vi "CLC_GEN4_L2_InPhaseCal_mW.vi"() -> ()   [LabVIEW 2023, in "Clover_Cell.lvlib"]
uses:
  Clover_Cell.lvlib
  lib/Anritsu Signal Analyzer Series/Anritsu Signal Analyzer Series.lvlib
  lib/ELTA/ELTA.lvlib
panel:
  in  "Daul_Ch_Phase_Sweep":bool
  in  "SweepSwitch?":u16(ring) items=["NoSweep(Single)", "Sweep"]
  in  "SweepMode":u16(ring) items=["Phase", "Gain"]
  in  "Method":u16(ring)=1 items=["dBm"=1, "mW"=2]
  in  "Polarity":u16(ring) items=["V", "H"]
  in  "VISA resource name":refnum<visa-resource-name>="TCPIP0::192.168.100.230::inst0::INSTR"
  in  "CenterFreq(GHz)":dbl=27.0
  in  "AvgTimes":i32=3
  in  "Single_Ch_Phase_Sweep":bool
  in  "TRXmode":u16(ring)=1 items=["Rx"=2, "Tx"=1]
  out "GainStep":i32=63
  out "PhaseStep":i32=63
  out "Channel":i32=63
  out "Total mW":dbl format="%.7f"
  out "Total dBm":dbl format="%.7f"
  out "Ref. mW":dbl format="%.7f"
  out "Ref. dBm":dbl format="%.7f"
  out "Main mW":dbl format="%.7f"
  out "Main dBm":dbl format="%.7f"
  out "Data":dbl[][](array[numeric])
  out "FileNAME_Single":string
  out "SA1":dbl[](graph)
  out "CurrentData":dbl[](array[numeric])
  out "Duration":dbl
  out "TotalTime":dbl format="%.2f"
  out "StopTime":timestamp=timestamp(3663835912.033212 s since 1904-01-01)
  out "FileNAME_Dual":string
  out "StartTime":timestamp=timestamp(3663835741.875155 s since 1904-01-01)
  out "TX/RX":u16=1
  out "error out":errorcluster
  out "output cluster":T1={"address"="192.168.100.111", "remote port or service name"=5025, "timeout ms (60000)"=10000}
  out "Operating \nChannel(s)":bool[][](array[boolean])
  out "OK?":bool
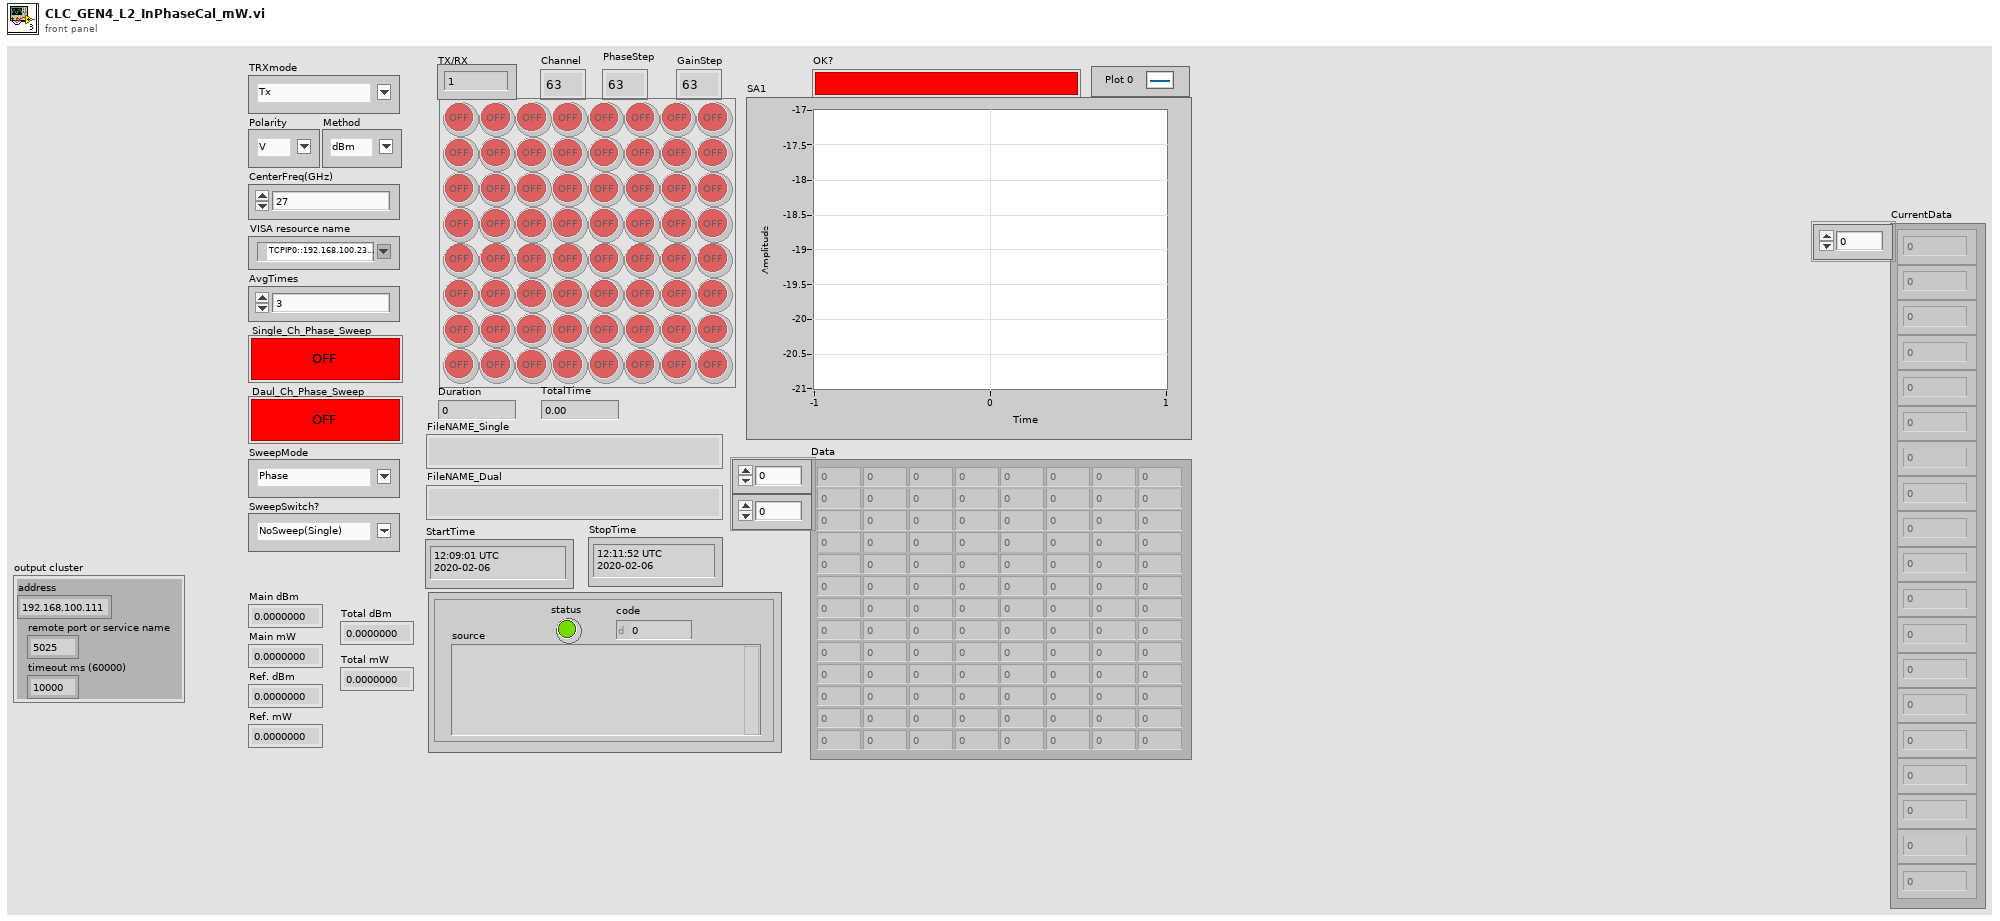
[diagram p1: front panel]
types:
  T1 = cluster{"address":string, "remote port or service name":u16, "timeout ms (60000)":i32}
  T2 = cluster{"Mode":u16, "Polarity":u16, "CH_ON/OFF":u16, "Channel":i32, "Gain":i32, "Phase":i32}
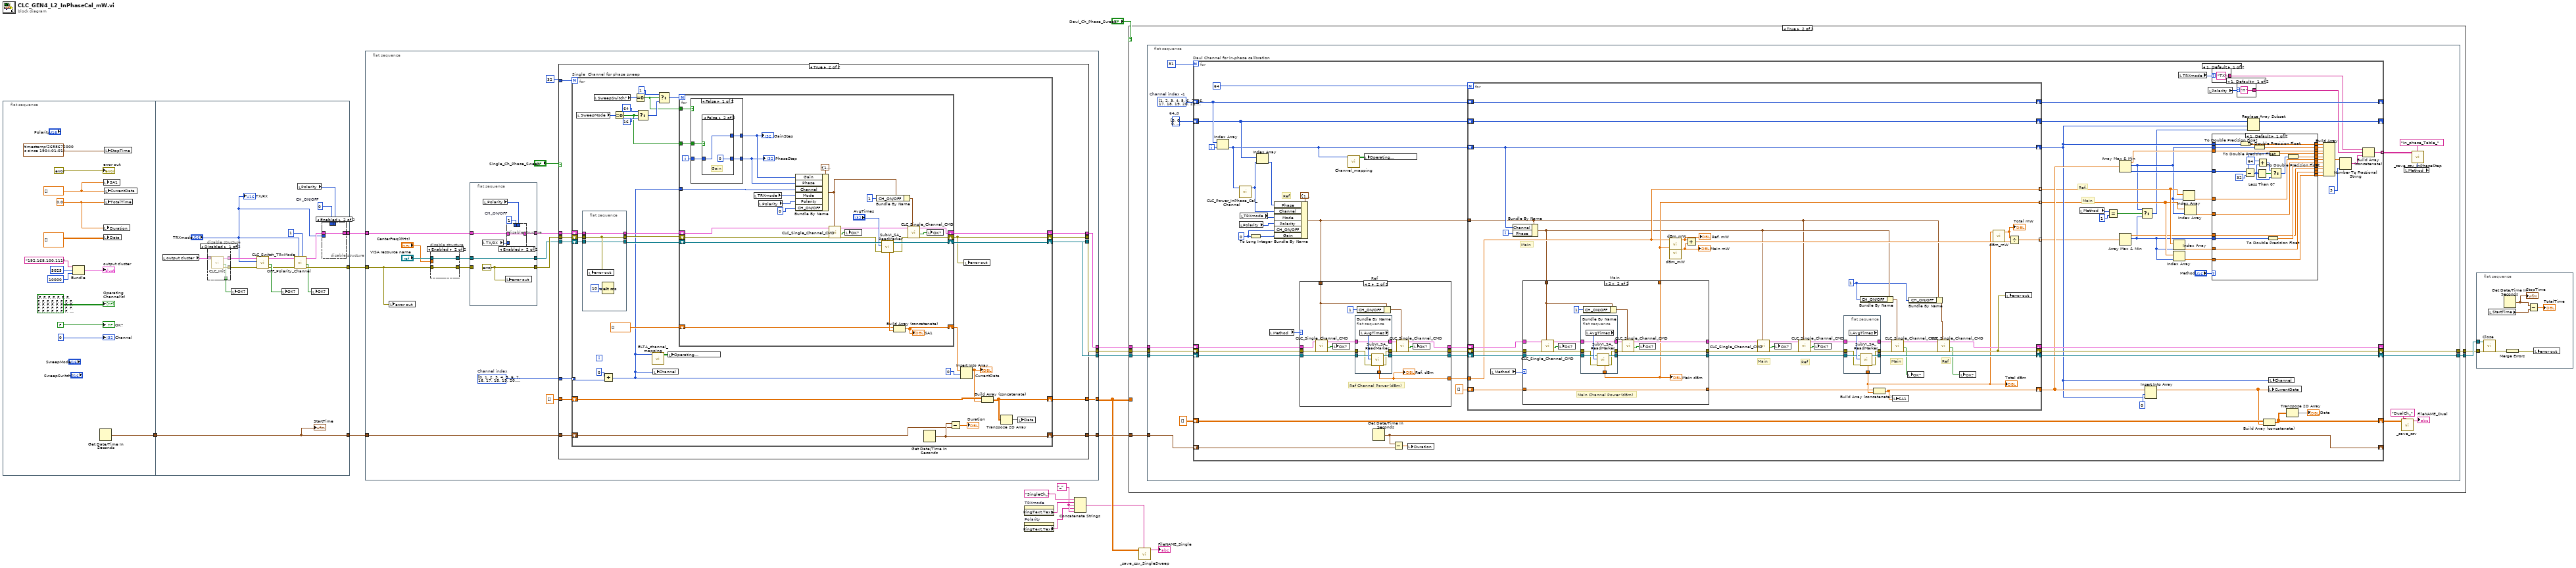
[diagram p0: block diagram]
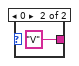
[diagram p3: hidden frame]
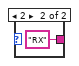
[diagram p4: hidden frame]
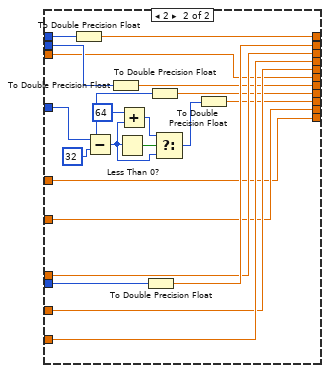
[diagram p5: hidden frame]
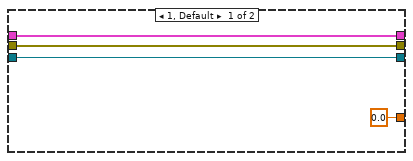
[diagram p6: hidden frame]
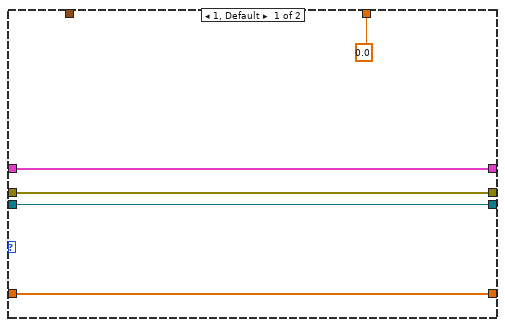
[diagram p7: hidden frame]
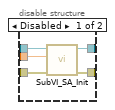
[diagram p8: hidden frame]
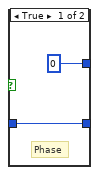
[diagram p10: hidden frame]
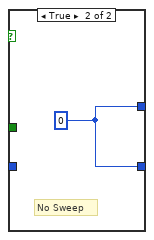
[diagram p11: hidden frame]
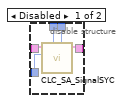
[diagram p12: hidden frame]
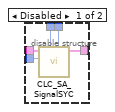
[diagram p13: hidden frame]
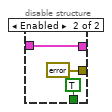
[diagram p14: hidden frame]
diagram:
  w2 = "_" ("delimiter (\\t)")
  n1 = flat-sequence {
    tunnel: [w19] -> w18
    tunnel: w18 -> [w35]
    tunnel: [w38] -> w9
    tunnel: [w42] -> w10
    tunnel: [w35] -> w17
    frame #0 {
      w23 = dbl[] []
      w26 = 0.0 ("TotalTime")
      n2 = Bundle("address"="192.168.100.111", "remote port or service name"=u16 5025, "timeout ms (60000)"=10000) -> (→"output cluster":T1)  [unwired: 1 in]
      n3 = Get Date/Time In Seconds() -> (seconds since 1Jan1904=w19:timestamp)
      n4 = local write "SA1"(w23) -> ()
      n5 = local write "Duration"(w26) -> ()
      n6 = local write "Data"(dbl[][] []) -> ()
      n7 = local write "StopTime"(timestamp(2658672000.001 s since 1904-01-01) ("StopTime")) -> ()
      n8 = local write "CurrentData"(w23) -> ()
      n9 = local write "TotalTime"(w26) -> ()
      "error out" <- errorcluster {"status"=FALSE, "code"=0, "source"=""} ("error out")
      "Operating \nChannel(s)" <- bool[][] [[FALSE, FALSE, FALSE, FALSE, FALSE, FALSE, FALSE, FALSE], [FALSE, FALSE, FALSE, FALSE, FALSE, FALSE, FALSE, FALSE], [FALSE, FALSE, FALSE, FALSE, FALSE, FALSE, FALSE, FALSE], [FALSE, FALSE, FALSE, FALSE, FALSE, FALSE, FALSE, FALSE], [FALSE, FALSE, FALSE, FALSE, FALSE, FALSE, FALSE, FALSE], [FALSE, FALSE, FALSE, FALSE, FALSE, FALSE, FALSE, FALSE], [FALSE, FALSE, FALSE, FALSE, FALSE, FALSE, FALSE, FALSE], [FALSE, FALSE, FALSE, FALSE, FALSE, FALSE, FALSE, FALSE]] ("Operating \nChannel(s)")
      "Channel" <- 0 ("Channel")
      "OK?" <- FALSE ("OK?")
    }
    frame #1 {
      w37 = u16 0  # CH_ON/OFF
      n10 = local read "output cluster"() -> (w47:T1)
      n11 = disable-structure shown="Disabled" {
        disable-tunnel: w47 -> [w57 w60]
        disable-tunnel: [w56 w60] -> w46
        disable-tunnel: [w55 errorcluster {"status"=FALSE, "code"=0, "source"=""} ("error in (no error)")] -> w44
        disable-tunnel: [w54 TRUE ("OK?")] -> w36
        frame Disabled {
          n12 = call "CLC_Init.vi"("TCPIPin"=w57) -> ("error out"=w55:errorcluster, "Status"=w54:bool, "TCPIPin 2"=w56:T1)  [unwired: 8 in]
        }
        frame Enabled {
        }
      }
      n13 = local write "OK?"(w36) -> ()
      n14 = call "CLC_Switch_TRxMode.vi"("error in (no error)"=w44, "Text Ring"="TRXmode", "TCPIPin"=w46) -> ("error out"=w43:errorcluster, "OK?"=w45:bool, "TCPIPin 2"=w41:T1)  [unwired: 6 in]
      n15 = local write "OK?"(w45) -> ()
      n16 = call "OFF_Polarity_Channel.vi"("CH_ON:0/OFF:1"=u16 1, "Mode"="TRXmode", "error in"=w43, "TCPIPin"=w41) -> ("error out"=w42:errorcluster, "OK?"=w40:bool, "TCPIPout"=w39:T1)  [unwired: 5 in]
      n17 = local read "Polarity"() -> (w33:u16)
      n18 = local write "OK?"(w40) -> ()
      n19 = disable-structure shown="Enabled" {
        disable-tunnel: w39 -> [w52 w53]
        disable-tunnel: [w51 w53] -> w38
        disable-tunnel: w37 -> [w50 _]
        disable-tunnel: w33 -> [w49 _]
        disable-tunnel: "TRXmode" -> [w48 _]
        frame Disabled {
          n20 = call "CLC_SA_SignalSYC.vi"("Polarity"=w49, "CH_ON/OFF"=w50, "Mode"=w48, "TCPIPin"=w52) -> ("TCPIPout"=w51:T1)  [unwired: 7 in]
        }
        frame Enabled {
        }
      }
      "StartTime" <- w35
      "TX/RX" <- "TRXmode"
    }
  }
  n21 = flat-sequence {
    tunnel: w17 -> [w77]
    tunnel: [w76] -> w16
    tunnel: [w75] -> w15
    tunnel: [w74] -> w14
    tunnel: [w73] -> w11
    tunnel: w10 -> [w71]
    tunnel: w9 -> [w66]
    tunnel: [w61] -> w6
    frame #0 {
      w68 = i32[] [0, 1, 2, 3, 4, 5, 6, 7, 16, 17, 18, 19, 20, 21, 22, 23, 32, 33, 34, 35, 36, 37, 38, 39, 48, 49, 50, 51, 52, 53, 54, 55]  # Channel index
      n22 = local write "error out"(w71) -> ()
      n23 = disable-structure shown="Enabled" {
        disable-tunnel: "VISA resource name" -> [w84 w86]
        disable-tunnel: [w83 w85] -> w72
        disable-tunnel: w71 -> [w82 w85]
        disable-tunnel: "CenterFreq(GHz)" -> [w81 _]
        disable-tunnel: [w80 w86] -> w65
        frame Disabled {
          n24 = call "SubVI_SA_Init.vi"("error in (no error)"=w82, "CenterFreq(GHz) 2"=w81, "VISA resource name"=w84) -> ("error out 2"=w83:errorcluster, "VISA resource name out"=w80:refnum<visa-resource-name>)  [unwired: 6 in, 1 out]
        }
        frame Enabled {
        }
      }
      n25 = flat-sequence {
        tunnel: w72 -> [_]
        tunnel: [w177] -> w67
        tunnel: w66 -> [w182]
        tunnel: w65 -> [w183]
        tunnel: [w183] -> w64
        tunnel: [w181] -> w63
        frame #0 {
          w177 = errorcluster {"status"=FALSE, "code"=0, "source"=""} ("error in (no error)")
          w180 = u16 1  # CH_ON/OFF
          n26 = local read "TX/RX"() -> (w178:u16)
          n27 = local read "Polarity"() -> (w179:u16)
          n28 = local write "error out"(w177) -> ()
          n29 = disable-structure shown="Enabled" {
            disable-tunnel: w182 -> [w188 w189]
            disable-tunnel: [w187 w189] -> w181
            disable-tunnel: w180 -> [w186 _]
            disable-tunnel: w179 -> [w185 _]
            disable-tunnel: w178 -> [w184 _]
            frame Disabled {
              n30 = call "CLC_SA_SignalSYC.vi"("Polarity"=w185, "CH_ON/OFF"=w186, "Mode"=w184, "TCPIPin"=w188) -> ("TCPIPout"=w187:T1)  [unwired: 7 in]
            }
            frame Enabled {
            }
          }
        }
      }
      n31 = case shown="True" "Single_Ch_Phase_Sweep" {
        tunnel: [w88 w103] -> w61
        tunnel: 32 -> [_ w102]
        tunnel: w77 -> [w87 w101]
        tunnel: [w89 w100] -> w76
        tunnel: [w90 w99] -> w75
        tunnel: [w91 w98] -> w74
        tunnel: [w87 w97] -> w73
        tunnel: dbl[][] [] -> [w88 w96]
        tunnel: w68 -> [_ w95]
        tunnel: w67 -> [w90 w94]
        tunnel: w64 -> [w89 w93]
        tunnel: w63 -> [w91 w92]
        frame False {
        }
        frame True {
          n32 = for "Single  Channel for phase sweep" {
            N: w102 -> [_]
            shift-right: [w135] -> w98
            shift-left: w92 -> [w120]
            shift-right: [w130] -> w99
            shift-left: w94 -> [w122]
            shift-right: [w134] -> w100
            shift-left: w93 -> [w119]
            shift-right: [w128] -> w103
            shift-left: w96 -> [w129]
            shift-right: [w132] -> w97
            shift-left: w101 -> [w131]
            tunnel: w95 -> [w116] mode=indexing
            n33 = local read "SweepMode"() -> (w112:u16)
            n34 = flat-sequence {
              tunnel: [w137] -> w118
              tunnel: w122 -> [w138]
              tunnel: [w138] -> w121
              tunnel: w120 -> [w137]
              tunnel: w119 -> [w136]
              tunnel: [w136] -> w117
              frame #0 {
                n35 = local write "error out"(w138) -> ()
                n36 = Wait (ms)(milliseconds to wait=u32 10) -> ()  [unwired: 1 out]
              }
            }
            n37 = local read "SweepSwitch?"() -> (w111:u16)
            n38 = Add(x=0, y=w116) -> (x+y=w113:i32)
            n39 = Equal To 0?(x=w112) -> (x = 0?=w104:bool)
            n40 = Equal To 0?(x=w111) -> (x = 0?=w105:bool)
            n41 = Select(t=64, s=w104, f=16) -> (s? t:f=w106:i32)
            n42 = call "ELTA_channel_mapping.vi"("Channel IN"=w113) -> ("Operating \nChannel(s)"=w114:bool[][])  [unwired: 10 in]
            n43 = local write "Channel"(w113) -> ()
            n44 = Select(t=1, s=w105, f=w106) -> (s? t:f=w109:i32)
            n45 = local write "Operating \nChannel(s)"(w114) -> ()
            n46 = for {
              N: w109 -> [_]
              shift-right: [w149] -> w135
              shift-left: w118 -> [w159]
              shift-right: [w151] -> w130
              shift-left: w121 -> [w161]
              shift-right: [w166] -> w134
              shift-left: w117 -> [w167]
              shift-right: [w162] -> w127
              shift-left: dbl[] [] -> [w163]
              tunnel: w113 -> [w156]
              tunnel: w105 -> [w144]
              tunnel: w104 -> [w141]
              i -> [w140]
              n47 = case shown="False" w144 {
                tunnel: [w168 w176] -> w143
                tunnel: [w169 w176] -> w142
                tunnel: w141 -> [w171 _]
                tunnel: w140 -> [w170 _]
                frame False {
                  n48 = case shown="False" w171 {
                    tunnel: w170 -> [w173 w174]
                    tunnel: [w173 0] -> w169
                    tunnel: [0 w174] -> w168
                    frame True {
                      # "Phase"
                    }
                    frame False {
                      # "Gain"
                    }
                  }
                }
                frame True {
                  w176 = 0
                  # "No Sweep"
                }
              }
              "PhaseStep" <- w142
              "GainStep" <- w143
              n49 = local read "TRXmode"() -> (w155:u16)
              n50 = local read "Polarity"() -> (w154:u16)
              n51 = Bundle By Name(cluster=T2 {"Mode"=1, "Polarity"=1, "CH_ON/OFF"=1, "Channel"=0, "Gain"=0, "Phase"=0} ("Channel params"), "Gain"=w143, "Phase"=w142, "Channel"=w156, "Mode"=w155, "Polarity"=w154, "CH_ON/OFF"=u16 0) -> (w148:T2)
              n52 = call "CLC_Single_Channel_CMD.vi"("Channel params"=w148, "error in"=w161, "TCPIPin"=w159) -> ("error out"=w160:errorcluster, "OK?"=w157:bool, "TCPIPout"=w150:T1)  [unwired: 6 in]
              n53 = local write "OK?"(w157) -> ()
              n54 = Bundle By Name(cluster=w148, "CH_ON/OFF"=u16 1) -> (w146:T2)
              n55 = call "SubVI_SA_ReadMarker.vi"("error in (no error)"=w160, "AvgTimes"="AvgTimes", "VISA resource name"=w167) -> ("error out"=w152:errorcluster, "VISA resource name out"=w166:refnum<visa-resource-name>, "Marker Power"=w164:dbl)  [unwired: 5 in, 1 out]
              n56 = Build Array (concatenate)(w163, w164) -> (w162:dbl[])
              "SA1" <- w162
              n57 = call "CLC_Single_Channel_CMD.vi"("Channel params"=w146, "error in"=w152, "TCPIPin"=w150) -> ("error out"=w151:errorcluster, "OK?"=w145:bool, "TCPIPout"=w149:T1)  [unwired: 6 in]
              n58 = local write "OK?"(w145) -> ()
            }
            n59 = Get Date/Time In Seconds() -> (seconds since 1Jan1904=w132:timestamp)
            n60 = Subtract(x=w132, y=w131) -> (x-y=→"Duration":dbl)
            n61 = Insert Into Array(array=w127, index=0, new element=w113) -> (w124:dbl[])
            "CurrentData" <- w124
            n62 = local write "error out"(w130) -> ()
            n63 = Build Array (concatenate)(w129, w124) -> (w128:dbl[][])
            n64 = Transpose 2D Array(2D array=w128) -> (transposed array=w115:dbl[][])
            n65 = local write "Data"(w115) -> ()
          }
        }
      }
    }
  }
  n66 = property on="TRXmode" class="Ring (strict)"() -> ("RingText.Text"=w4:string)  [unwired: 2 in, 2 out]
  n67 = property on="Polarity" class="Ring (strict)"() -> ("RingText.Text"=w1:string)  [unwired: 2 in, 2 out]
  n68 = Concatenate Strings("SingleCh_" ("delimiter (\\t)"), w4, w2, w1, w2) -> (w3:string)
  n69 = case shown="True" "Daul_Ch_Phase_Sweep" {
    tunnel: w16 -> [w191 w197]
    tunnel: w15 -> [w190 w196]
    tunnel: w14 -> [_ w195]
    tunnel: [w191 w194] -> w13
    tunnel: [w190 w193] -> w12
    tunnel: w11 -> [_ w192]
    tunnel: w6 -> [_ _]
    frame False {
    }
    frame True {
      n70 = flat-sequence {
        tunnel: w197 -> [w212]
        tunnel: w196 -> [w211]
        tunnel: w195 -> [w210]
        tunnel: [w209] -> w194
        tunnel: [w208] -> w193
        tunnel: w192 -> [w207]
        frame #0 {
          w204 = i32[] [0, 0, 0, 0, 0, 0, 0, 0, 0, 0, 0, 0, 0, 0, 0, 0, 0, 0, 0, 0, 0, 0, 0, 0, 0, 0, 0, 0, 0, 0, 0, 0, 0, 0, 0, 0, 0, 0, 0, 0, 0, 0, 0, 0, 0, 0, 0, 0, 0, 0, 0, 0, 0, 0, 0, 0, 0, 0, 0, 0, 0, 0, 0, 0]  # 64_0
          w205 = i32[] [1, 2, 3, 4, 5, 6, 7, 16, 17, 18, 19, 20, 21, 22, 23, 32, 33, 34, 35, 36, 37, 38, 39, 48, 49, 50, 51, 52, 53, 54, 55]  # Channel index -1
          n71 = for "Daul Channel for in-phase calibration" {
            N: 31 -> [_]
            shift-right: [w288] -> _
            shift-left: w210 -> [w249]
            shift-right: [w285] -> w208
            shift-left: w211 -> [w253]
            shift-right: [w286] -> w209
            shift-left: w212 -> [w251]
            shift-right: [w280] -> w199
            shift-left: dbl[][] [] -> [w281]
            shift-right: [w284] -> _
            shift-left: w207 -> [w283]
            shift-right: [w271] -> _
            shift-left: w204 -> [w246]
            tunnel: [w214] -> w200 mode=indexing
            shift-right: [w273] -> _
            shift-left: w205 -> [w272]
            i -> [w274]
            w255 = u16 0 ("CH_ON/OFF")
            # "Main"
            # "Ref."
            # "Ref"
            n72 = Index Array(array=w272, index=w274) -> (element=w242:i32)
            n73 = call "CLC_Power_InPhase_Cal_Channel.vi"("Channel IN"=w242) -> ("Ref_Channel"=w241:i32)  [unwired: 8 in, 2 out]
            n74 = local read "Polarity"() -> (w256:u16)
            n75 = local read "TRXmode"() -> (w257:u16)
            n76 = To Long Integer(number=w255) -> (32bit integer=w254:i32)
            n77 = Index Array(array=w246, index=w241) -> (element=w245:i32)
            n78 = local read "Method"() -> (w243:u16)
            n79 = Bundle By Name(cluster=T2 {"Mode"=1, "Polarity"=1, "CH_ON/OFF"=1, "Channel"=0, "Gain"=0, "Phase"=0} ("Channel params"), "Phase"=w245, "Channel"=w241, "Mode"=w257, "Polarity"=w256, "CH_ON/OFF"=w255, "Gain"=w254) -> (w244:T2)
            n80 = case "Ref" shown="2" w243 {
              tunnel: w253 -> [w337 w346]
              tunnel: [w337 w345] -> w252
              tunnel: w251 -> [w336 w344]
              tunnel: [w336 w343] -> w250
              tunnel: w249 -> [w338 w342]
              tunnel: [w338 w341] -> w248
              tunnel: [0.0 ("Marker Response") w340] -> w247
              tunnel: w244 -> [_ w339]
              frame 1, Default {
              }
              frame 2 {
                # "Ref Channel Power (dBm)"
                n81 = call "CLC_Single_Channel_CMD.vi"("Channel params"=w339, "error in"=w346, "TCPIPin"=w342) -> ("error out"=w353:errorcluster, "OK?"=w354:bool, "TCPIPout"=w352:T1)  [unwired: 6 in]
                n82 = local write "OK?"(w354) -> ()
                n83 = flat-sequence {
                  tunnel: [w361] -> w343
                  tunnel: [w359] -> w340
                  tunnel: w344 -> [w358]
                  tunnel: w353 -> [w357]
                  tunnel: [w356] -> w348
                  tunnel: w352 -> [w356]
                  tunnel: [w355] -> w349
                  frame #0 {
                    n84 = local read "AvgTimes"() -> (w360:i32)
                    n85 = call "SubVI_SA_ReadMarker.vi"("error in (no error)"=w357, "AvgTimes"=w360, "VISA resource name"=w358) -> ("error out"=w355:errorcluster, "VISA resource name out"=w361:refnum<visa-resource-name>, "Marker Power"=w359:dbl)  [unwired: 5 in, 1 out]
                  }
                }
                n86 = Bundle By Name(cluster=w339, "CH_ON/OFF"=u16 1) -> (w350:T2)
                n87 = call "CLC_Single_Channel_CMD.vi"("Channel params"=w350, "error in"=w349, "TCPIPin"=w348) -> ("error out"=w345:errorcluster, "OK?"=w351:bool, "TCPIPout"=w341:T1)  [unwired: 6 in]
                n88 = local write "OK?"(w351) -> ()
                "Ref. dBm" <- w340
              }
            }
            n89 = call "Channel_mapping.vi"("Channel IN"=w242) -> ("Operating \nChannel(s)"=w259:bool[][])  [unwired: 10 in]
            n90 = local write "Operating \nChannel(s)"(w259) -> ()
            n91 = Get Date/Time In Seconds() -> (seconds since 1Jan1904=w284:timestamp)
            n92 = Subtract(x=w284, y=w283) -> (x-y=w282:dbl)
            n93 = local write "Duration"(w282) -> ()
            n94 = for {
              N: 64 -> [_]
              shift-right: [w388] -> w288
              shift-left: w248 -> [w370]
              shift-right: [w392] -> w285
              shift-left: w252 -> [w383]
              shift-right: [w403] -> w286
              shift-left: w250 -> [w382]
              shift-right: [w385] -> w275
              shift-left: dbl[] [] -> [w372]
              shift-right: [w397] -> w270
              shift-left: w246 -> [w397]
              shift-right: [w387] -> w273
              shift-left: w272 -> [w387]
              shift-right: [w365] -> w269
              shift-left: w242 -> [w365]
              tunnel: [w369] -> w262 mode=indexing
              tunnel: [w376] -> w261 mode=indexing
              tunnel: [w377] -> w268 mode=indexing
              tunnel: w244 -> [w363]
              tunnel: w247 -> [w369]
              i -> [w366]
              w362 = u16 1 ("CH_ON/OFF")
              # "Main"
              # "Ref"
              # "Main"
              # "Ref"
              # "Main"
              n95 = local read "Method"() -> (w373:u16)
              n96 = Bundle By Name(cluster=w363, "Channel"=w365, "Phase"=w366) -> (w364:T2)
              n97 = case "Main" shown="2" w373 {
                tunnel: w383 -> [w406 w412]
                tunnel: w370 -> [w407 w413]
                tunnel: w382 -> [w405 w411]
                tunnel: [w407 w417] -> w381
                tunnel: [w406 w416] -> w380
                tunnel: [w405 w415] -> w379
                tunnel: w364 -> [_ w414]
                tunnel: [0.0 ("Marker Response") w409] -> w376
                tunnel: w372 -> [w404 w410]
                tunnel: [w404 w410] -> w371
                frame 1, Default {
                }
                frame 2 {
                  # "Main Channel Power (dBm)"
                  n98 = call "CLC_Single_Channel_CMD.vi"("Channel params"=w414, "error in"=w412, "TCPIPin"=w413) -> ("error out"=w419:errorcluster, "OK?"=w418:bool, "TCPIPout"=w420:T1)  [unwired: 6 in]
                  n99 = local write "OK?"(w418) -> ()
                  n100 = flat-sequence {
                    tunnel: [w432] -> w415
                    tunnel: [w430] -> w409
                    tunnel: w411 -> [w429]
                    tunnel: w419 -> [w428]
                    tunnel: [w427] -> w425
                    tunnel: w420 -> [w427]
                    tunnel: [w426] -> w424
                    frame #0 {
                      n101 = local read "AvgTimes"() -> (w431:i32)
                      n102 = call "SubVI_SA_ReadMarker.vi"("error in (no error)"=w428, "AvgTimes"=w431, "VISA resource name"=w429) -> ("error out"=w426:errorcluster, "VISA resource name out"=w432:refnum<visa-resource-name>, "Marker Power"=w430:dbl)  [unwired: 5 in, 1 out]
                    }
                  }
                  n103 = Bundle By Name(cluster=w414, "CH_ON/OFF"=u16 1) -> (w423:T2)
                  n104 = call "CLC_Single_Channel_CMD.vi"("Channel params"=w423, "error in"=w424, "TCPIPin"=w425) -> ("error out"=w416:errorcluster, "OK?"=w421:bool, "TCPIPout"=w417:T1)  [unwired: 6 in]
                  n105 = local write "OK?"(w421) -> ()
                  "Main dBm" <- w409
                }
              }
              n106 = call "dBm_mW.vi"("dBm"=w369) -> ("mW"=w368:dbl)  [unwired: 10 in]
              "Ref. mW" <- w368
              n107 = call "dBm_mW.vi"("dBm"=w376) -> ("mW"=w367:dbl)  [unwired: 10 in]
              "Main mW" <- w367
              n108 = Add(x=w368, y=w367) -> (x+y=w378:dbl)
              n109 = call "CLC_Single_Channel_CMD.vi"("Channel params"=w364, "error in"=w380, "TCPIPin"=w381) -> ("error out"=w401:errorcluster, "OK?"=w400:bool, "TCPIPout"=w402:T1)  [unwired: 6 in]
              n110 = local write "OK?"(w400) -> ()
              n111 = call "CLC_Single_Channel_CMD.vi"("Channel params"=w363, "error in"=w401, "TCPIPin"=w402) -> ("error out"=w398:errorcluster, "OK?"=w399:bool, "TCPIPout"=w396:T1)  [unwired: 6 in]
              n112 = local write "OK?"(w399) -> ()
              n113 = flat-sequence {
                tunnel: [w439] -> w403
                tunnel: [w437] -> w375
                tunnel: w379 -> [w436]
                tunnel: w398 -> [w435]
                tunnel: [w434] -> w395
                tunnel: w396 -> [w434]
                tunnel: [w433] -> w384
                frame #0 {
                  n114 = local read "AvgTimes"() -> (w438:i32)
                  n115 = call "SubVI_SA_ReadMarker.vi"("error in (no error)"=w435, "AvgTimes"=w438, "VISA resource name"=w436) -> ("error out"=w433:errorcluster, "VISA resource name out"=w439:refnum<visa-resource-name>, "Marker Power"=w437:dbl)  [unwired: 5 in, 1 out]
                }
              }
              n116 = Bundle By Name(cluster=w364, "CH_ON/OFF"=w362) -> (w386:T2)
              n117 = Build Array (concatenate)(w371, w375) -> (w385:dbl[])
              n118 = call "CLC_Single_Channel_CMD.vi"("Channel params"=w386, "error in"=w384, "TCPIPin"=w395) -> ("error out"=w393:errorcluster, "OK?"=w394:bool, "TCPIPout"=w391:T1)  [unwired: 6 in]
              n119 = local write "SA1"(w385) -> ()
              n120 = local write "OK?"(w394) -> ()
              n121 = Bundle By Name(cluster=w363, "CH_ON/OFF"=w362) -> (w390:T2)
              n122 = call "CLC_Single_Channel_CMD.vi"("Channel params"=w390, "error in"=w393, "TCPIPin"=w391) -> ("error out"=w392:errorcluster, "OK?"=w389:bool, "TCPIPout"=w388:T1)  [unwired: 6 in]
              n123 = local write "OK?"(w389) -> ()
              n124 = call "dBm_mW.vi"("dBm"=w375) -> ("mW"=w374:dbl)  [unwired: 10 in]
              "Total mW" <- w374
              n125 = local write "error out"(w392) -> ()
              n126 = Divide(x=w374, y=w378) -> (x/y=w377:dbl)
              "Total dBm" <- w375
            }
            n127 = local read "Method"() -> (w228:u16)
            n128 = Equal?(x=w228, y=u16 1) -> (x = y?=w226:bool)
            n129 = Array Max & Min(array=w275) -> (max value=w238:dbl, max index (indices)=w225:i32, min index (indices)=w260:i32)  [unwired: 1 out]
            n130 = Array Max & Min(array=w268) -> (max value=w232:dbl, max index (indices)=w224:i32)  [unwired: 2 out]
            n131 = Select(t=w225, s=w226, f=w224) -> (s? t:f=w223:i32)
            n132 = Insert Into Array(array=w275, index=0, new element=w269) -> (w276:dbl[])
            n133 = Index Array(array=w262, index=w224) -> (element=w231:dbl)
            n134 = Index Array(array=w261, index=w224) -> (element=w230:dbl)
            n135 = local read "TRXmode"() -> (w219:u16)
            n136 = Index Array(array=w262, index=w225) -> (element=w236:dbl)
            n137 = Index Array(array=w261, index=w225) -> (element=w235:dbl)
            n138 = local read "Polarity"() -> (w218:u16)
            n139 = case shown="1, Default" w219 {
              tunnel: ["TX" "RX"] -> w215
              frame 1, Default {
              }
              frame 2 {
              }
            }
            n140 = case shown="1, Default" "Method" {
              tunnel: w269 -> [w307 w328]
              tunnel: [w293 w322] -> w267
              tunnel: [w306 w321] -> w266
              tunnel: [w305 w320] -> w265
              tunnel: [w304 w324] -> w264
              tunnel: [w303 w317] -> w263
              tunnel: w260 -> [w302 w327]
              tunnel: w224 -> [w301 w326]
              tunnel: w225 -> [w300 w325]
              tunnel: w238 -> [w293 w319]
              tunnel: [w294 w323] -> w239
              tunnel: [w299 w319] -> w237
              tunnel: w236 -> [w299 w314]
              tunnel: w235 -> [w298 w315]
              tunnel: [w298 w318] -> w234
              tunnel: [w297 w316] -> w233
              tunnel: w232 -> [w297 w322]
              tunnel: w231 -> [w296 w320]
              tunnel: w230 -> [w295 w321]
              tunnel: [w295 w314] -> w229
              tunnel: [w296 w315] -> w222
              frame 1, Default {
                n141 = To Double Precision Float(number=w307) -> (double precision float=w304:dbl)
                n142 = Subtract(x=w302, y=32) -> (x-y=w309:i32)
                n143 = To Double Precision Float(number=w300) -> (double precision float=w294:dbl)
                n144 = Less Than 0?(x=w309) -> (x < 0?=w312:bool)
                n145 = Add(x=64, y=w309) -> (x+y=w310:i32)
                n146 = To Double Precision Float(number=w301) -> (double precision float=w303:dbl)
                n147 = To Double Precision Float(number=w302) -> (double precision float=w306:dbl)
                n148 = Select(t=w310, s=w312, f=w309) -> (s? t:f=w308:i32)
                n149 = To Double Precision Float(number=w308) -> (double precision float=w305:dbl)
              }
              frame 2 {
                n150 = To Double Precision Float(number=w328) -> (double precision float=w324:dbl)
                n151 = Subtract(x=w327, y=32) -> (x-y=w330:i32)
                n152 = To Double Precision Float(number=w325) -> (double precision float=w318:dbl)
                n153 = Less Than 0?(x=w330) -> (x < 0?=w333:bool)
                n154 = Add(x=64, y=w330) -> (x+y=w331:i32)
                n155 = To Double Precision Float(number=w326) -> (double precision float=w323:dbl)
                n156 = To Double Precision Float(number=w327) -> (double precision float=w317:dbl)
                n157 = Select(t=w331, s=w333, f=w330) -> (s? t:f=w329:i32)
                n158 = To Double Precision Float(number=w329) -> (double precision float=w316:dbl)
              }
            }
            n159 = case shown="1, Default" w218 {
              tunnel: ["H" "V"] -> w216
              frame 1, Default {
              }
              frame 0 {
              }
            }
            n160 = Replace Array Subset(array=w270, new element=w223, index=w269) -> (w271:i32[])
            n161 = Build Array (concatenate)(w281, w276) -> (w280:dbl[][])
            n162 = local write "CurrentData"(w276) -> ()
            n163 = local write "Channel"(w269) -> ()
            n164 = Transpose 2D Array(2D array=w280) -> (transposed array=→"Data":dbl[][])
            n165 = Build Array(w264, w239, w267, w266, w265, w237, w234, w263, w233, w222, w229) -> (w220:dbl[])
            n166 = Number To Fractional String(number=w220, precision (6)=i16 3) -> (F-format string=w217:string[])  [unwired: 2 in]
            n167 = Build Array (concatenate)(w215, w216, w217) -> (w214:string[])
          }
          n168 = call "_save_csv.vi"("delimiter (\\t)"="DualCh_" ("delimiter (\\t)"), "Data"=w199) -> ("FileName"=→"FileNAME_Dual":string)  [unwired: 9 in]
          n169 = local read "Method"() -> (w198:u16)
          n170 = call "_save_csv_InPhaseStep.vi"("Method"=w198, "delimiter (\\t)"="In_phase_Table_" ("delimiter (\\t)"), "dataInput"=w200) -> ()  [unwired: 8 in, 1 out]
        }
      }
    }
  }
  n171 = call "_save_csv_SingleSweep.vi"("delimiter (\\t)"=w3, "Data"=w6) -> ("FileName"=→"FileNAME_Single":string)  [unwired: 9 in]
  n172 = flat-sequence {
    tunnel: w13 -> [w445]
    tunnel: w12 -> [w444]
    frame #0 {
      n173 = call "Close.vi"("error in (no error)"=w444, "VISA resource name"=w445) -> ("error out"=w446:errorcluster)  [unwired: 9 in]
      n174 = local read "StartTime"() -> (w440:timestamp)
      n175 = Get Date/Time In Seconds() -> (seconds since 1Jan1904=w441:timestamp)
      "StopTime" <- w441
      n176 = Merge Errors(w446) -> (w443:errorcluster)
      n177 = Subtract(x=w441, y=w440) -> (x-y=→"TotalTime":dbl)
      n178 = local write "error out"(w443) -> ()
    }
  }
